vi "EXA shm issue Command exit Control LV.vi"(8 "error in (no error)":errorcluster, 11 "command_exitControl_Ctl":cluster{"state":u8}) -> (0 "error out":errorcluster, 2 "function return":i32, 3 "command_exitControl_Ctl out":cluster{"state":u8})   [LabVIEW 2016, in "SALLV_EXA.lvlib"]
doc: "int EXA_shm_issueCommand_exitControlLV(EXA_command_exitControlLV *command_exitControl_Ctl );"
uses:
  SALLV_EXA.lvlib
  SALLV_EXA.so
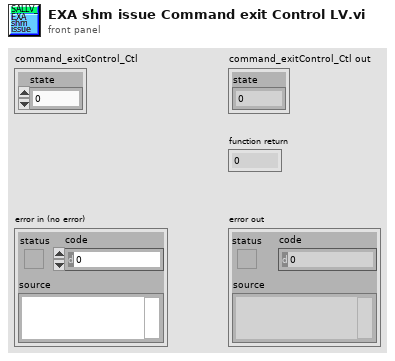
[diagram p1: front panel]
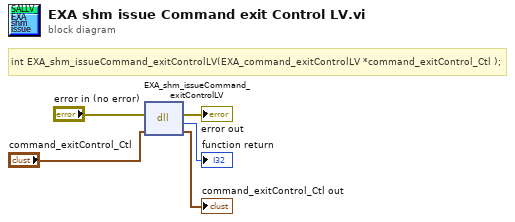
[diagram p0: block diagram]
diagram:
  # "int EXA_shm_issueCommand_exitControlLV(EXA_command_exitControlLV *command_exitControl_Ctl );"
  n1 = dll-call lib="home/plotz/SALLV_EXA/SALLV_EXA.*" fn="EXA_shm_issueCommand_exitControlLV"(error in="error in (no error)", "command_exitControl_Ctl"="command_exitControl_Ctl") -> (error out=→"error out":errorcluster, →"function return":i32, "command_exitControl_Ctl"=→"command_exitControl_Ctl out":cluster{"state":u8})  [unwired: 2 in, 1 out]
